vi "ABB Calc Brg dT.vi"(10 "Primary coolant":u16, 11 "Readings in":dbl[][](array[numeric])) -> (0 "dT (deg/hr)":dbl, 2 "NDE rise":dbl, 3 "DE rise":dbl, 4 "run time":dbl, 5 "lastindex":i32)   [LabVIEW 2017]
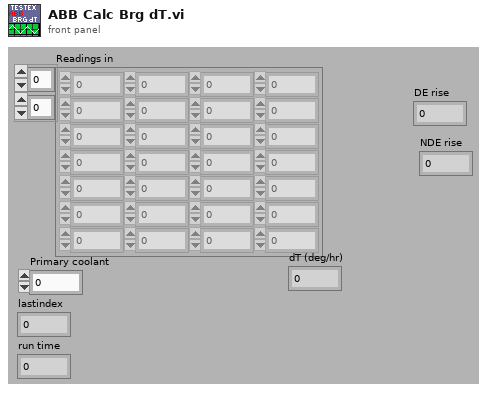
[diagram p1: front panel]
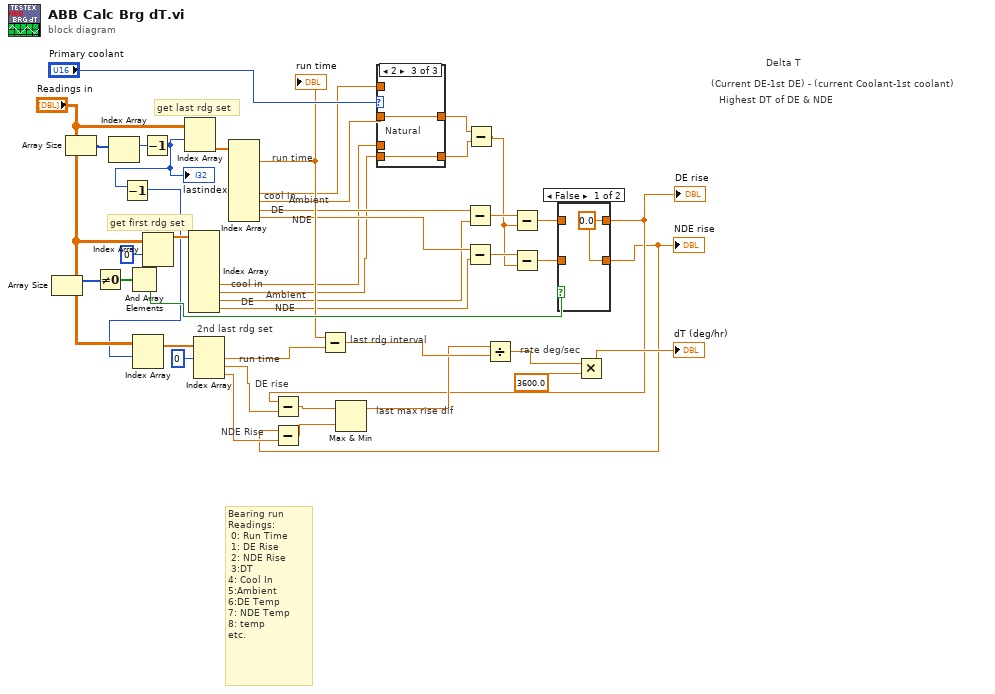
[diagram p0: block diagram]
diagram:
  # "NDE Rise"
  # "Bearing run Readings:\n 0: Run Time\n 1: DE Rise\n 2: NDE Rise\n 3:DT\n4: Cool In\n5:Ambient\n6:DE Temp\n7: NDE Temp\n8: temp\netc."
  # "rate deg/sec"
  # "last max rise dif"
  # "DE rise"
  # "run time"
  # "run time"
  # "last rdg interval"
  # "2nd last rdg set"
  # "NDE"
  # "DE"
  # "Ambient"
  # "cool in"
  # "NDE"
  # "DE"
  # "Ambient"
  # "cool in"
  # "get first rdg set"
  # "Delta T"
  # "Highest DT of DE & NDE"
  # "(Current DE-1st DE) - (current Coolant-1st coolant)"
  # "get last rdg set"
  n1 = Array Size(array="Readings in") -> (size(s)=w31:i32[])
  n2 = Array Size(array="Readings in") -> (size(s)=w42:i32[])
  n3 = Not Equal To 0?(x=w31) -> (x != 0?=w30:bool[])
  n4 = Index Array(array=w42) -> (element=w41:i32)  [unwired: 1 in]
  n5 = And Array Elements(Boolean array=w30) -> (logical AND=w29:bool)
  n6 = Decrement(x=w41) -> (x-1=w26:i32)
  "lastindex" <- w26
  n7 = Decrement(x=w26) -> (x-1=w23:i32)
  n8 = Index Array(array="Readings in", index (row)=w23) -> (element=w25:dbl[])  [unwired: 1 in]
  n9 = Index Array(array="Readings in", index (row)=0) -> (element=w39:dbl[])  [unwired: 1 in]
  n10 = Index Array(array="Readings in", index (row)=w26) -> (element=w38:dbl[])  [unwired: 1 in]
  n11 = Index Array(array=w39) -> (element #5=w9:dbl, element #6=w10:dbl, element #7=w11:dbl, element #8=w12:dbl)  [unwired: 8 in, 4 out]
  n12 = Index Array(array=w25, index #1=0 ("index")) -> (element #1=w21:dbl, element #2=w4:dbl, element #3=w2:dbl)  [unwired: 2 in]
  n13 = Index Array(array=w38) -> (element #1=w22:dbl, element #5=w13:dbl, element #6=w14:dbl, element #7=w15:dbl, element #8=w16:dbl)  [unwired: 8 in, 3 out]
  "run time" <- w22
  n14 = Subtract(x=w22, y=w21) -> (x-y=w20:dbl)
  n15 = case shown="2" "Primary coolant" {
    tunnel: w14 -> [_ _ w48]
    tunnel: [w44 w46 w48] -> w34
    tunnel: w13 -> [w44 w46 _]
    tunnel: w10 -> [_ _ w47]
    tunnel: w9 -> [w43 w45 _]
    tunnel: [w43 w45 w47] -> w33
    frame 0, Default {
      # "Oil"
    }
    frame 1 {
      # "Water"
    }
    frame 2 {
      # "Natural"
    }
  }
  n16 = Subtract(x=w15, y=w11) -> (x-y=w37:dbl)
  n17 = Subtract(x=w16, y=w12) -> (x-y=w36:dbl)
  n18 = Subtract(x=w34, y=w33) -> (x-y=w32:dbl)
  n19 = Subtract(x=w37, y=w32) -> (x-y=w28:dbl)
  n20 = Subtract(x=w36, y=w32) -> (x-y=w27:dbl)
  n21 = case shown="False" w29 {
    tunnel: w28 -> [_ w51]
    tunnel: [w49 w51] -> w3
    tunnel: w27 -> [_ w50]
    tunnel: [w49 w50] -> w1
    frame False {
      w49 = 0.0
    }
    frame True {
    }
  }
  "DE rise" <- w3
  "NDE rise" <- w1
  n22 = Subtract(x=w3, y=w4) -> (x-y=w7:dbl)
  n23 = Subtract(x=w1, y=w2) -> (x-y=w6:dbl)
  n24 = Max & Min(x=w7, y=w6) -> (max(x,y)=w5:dbl)  [unwired: 1 out]
  n25 = Divide(x=w5, y=w20) -> (x/y=w18:dbl)
  n26 = Multiply(x=w18, y=3600.0) -> (x*y=→"dT (deg/hr)":dbl)
